vi "启动条件判断.vi"(7 "时间源":T1, 8 "仪器状态":bool, 9 "启动次数":i32, 10 "间隔计时":i32, 11 "周期设置输出":T6={"周期模式"=enum."不启用", "定点周期"={"启动命令"=0, "启动命令 2"=0, "启动命令 3"=0, "启动命令 4"=0, "启动命令 5"=0, "启动命令 6"=0, "启动命令 7"=0, "启动命令 8"=0, "启动命令 9"=0, "启动命令 10"=0, "启动命令 11"=0, "启动命令 12"=0, "启动命令 13"=0, "启动命令 14"=0, "启动命令 15"=0, "启动命令 16"=0, "启动命令 17"=0, "启动命令 18"=0, "启动命令 19"=0, "启动命令 20"=0, "启动命令 21"=0, "启动命令 22"=0, "启动命令 23"=0, "启动命令 24"=0}, "间隔设置"={"启动命令"=0, "启动间隔"=0.0, "启动次数"=0}, "测量参数"={"氨氮"=TRUE, "总磷"=TRUE, "总氮"=TRUE, "CODMn"=TRUE, "CODCr"=TRUE}} {"定点周期"."启动命令 24" items=["", "加标回收（启动采配水）", "加标回收（不启动采配水）", "水样测试（启动采配水）", "水样测试（不启动采配水）"]; "定点周期"."启动命令 23" items=["", "加标回收（启动采配水）", "加标回收（不启动采配水）", "水样测试（启动采配水）", "水样测试（不启动采配水）"]; "定点周期"."启动命令 22" items=["", "加标回收（启动采配水）", "加标回收（不启动采配水）", "水样测试（启动采配水）", "水样测试（不启动采配水）"]; "定点周期"."启动命令 21" items=["", "加标回收（启动采配水）", "加标回收（不启动采配水）", "水样测试（启动采配水）", "水样测试（不启动采配水）"]; "定点周期"."启动命令 20" items=["", "加标回收（启动采配水）", "加标回收（不启动采配水）", "水样测试（启动采配水）", "水样测试（不启动采配水）"]; "定点周期"."启动命令 19" items=["", "加标回收（启动采配水）", "加标回收（不启动采配水）", "水样测试（启动采配水）", "水样测试（不启动采配水）"]; "定点周期"."启动命令 18" items=["", "加标回收（启动采配水）", "加标回收（不启动采配水）", "水样测试（启动采配水）", "水样测试（不启动采配水）"]; "定点周期"."启动命令 17" items=["", "加标回收（启动采配水）", "加标回收（不启动采配水）", "水样测试（启动采配水）", "水样测试（不启动采配水）"]; "定点周期"."启动命令 16" items=["", "加标回收（启动采配水）", "加标回收（不启动采配水）", "水样测试（启动采配水）", "水样测试（不启动采配水）"]; "定点周期"."启动命令 15" items=["", "加标回收（启动采配水）", "加标回收（不启动采配水）", "水样测试（启动采配水）", "水样测试（不启动采配水）"]; "定点周期"."启动命令 14" items=["", "加标回收（启动采配水）", "加标回收（不启动采配水）", "水样测试（启动采配水）", "水样测试（不启动采配水）"]; "定点周期"."启动命令 13" items=["", "加标回收（启动采配水）", "加标回收（不启动采配水）", "水样测试（启动采配水）", "水样测试（不启动采配水）"]; "定点周期"."启动命令 12" items=["", "加标回收（启动采配水）", "加标回收（不启动采配水）", "水样测试（启动采配水）", "水样测试（不启动采配水）"]; "定点周期"."启动命令 11" items=["", "加标回收（启动采配水）", "加标回收（不启动采配水）", "水样测试（启动采配水）", "水样测试（不启动采配水）"]; "定点周期"."启动命令 10" items=["", "加标回收（启动采配水）", "加标回收（不启动采配水）", "水样测试（启动采配水）", "水样测试（不启动采配水）"]; "定点周期"."启动命令 9" items=["", "加标回收（启动采配水）", "加标回收（不启动采配水）", "水样测试（启动采配水）", "水样测试（不启动采配水）"]; "定点周期"."启动命令 8" items=["", "加标回收（启动采配水）", "加标回收（不启动采配水）", "水样测试（启动采配水）", "水样测试（不启动采配水）"]; "定点周期"."启动命令 7" items=["", "加标回收（启动采配水）", "加标回收（不启动采配水）", "水样测试（启动采配水）", "水样测试（不启动采配水）"]; "定点周期"."启动命令 6" items=["", "加标回收（启动采配水）", "加标回收（不启动采配水）", "水样测试（启动采配水）", "水样测试（不启动采配水）"]; "定点周期"."启动命令 5" items=["", "加标回收（启动采配水）", "加标回收（不启动采配水）", "水样测试（启动采配水）", "水样测试（不启动采配水）"]; "定点周期"."启动命令 4" items=["", "加标回收（启动采配水）", "加标回收（不启动采配水）", "水样测试（启动采配水）", "水样测试（不启动采配水）"]; "定点周期"."启动命令 3" items=["", "加标回收（启动采配水）", "加标回收（不启动采配水）", "水样测试（启动采配水）", "水样测试（不启动采配水）"]; "定点周期"."启动命令 2" items=["", "加标回收（启动采配水）", "加标回收（不启动采配水）", "水样测试（启动采配水）", "水样测试（不启动采配水）"]; "定点周期"."启动命令" items=["", "加标回收（启动采配水）", "加标回收（不启动采配水）", "水样测试（启动采配水）", "水样测试（不启动采配水）"]; "间隔设置"."启动命令" items=["", "加标回收（启动采配水）", "加标回收（不启动采配水）", "水样测试（启动采配水）", "水样测试（不启动采配水）"]}) -> (2 "重新配置":bool, 3 "Data":T7={"启动"=FALSE, "控制命令"=enum."加标回收（启动采配水）", "测量参数"={"氨氮"=TRUE, "总磷"=TRUE, "总氮"=TRUE, "CODMn"=TRUE, "CODCr"=TRUE}} caption="数据")   [LabVIEW 2016, in "ZK定时设置.xctl"]
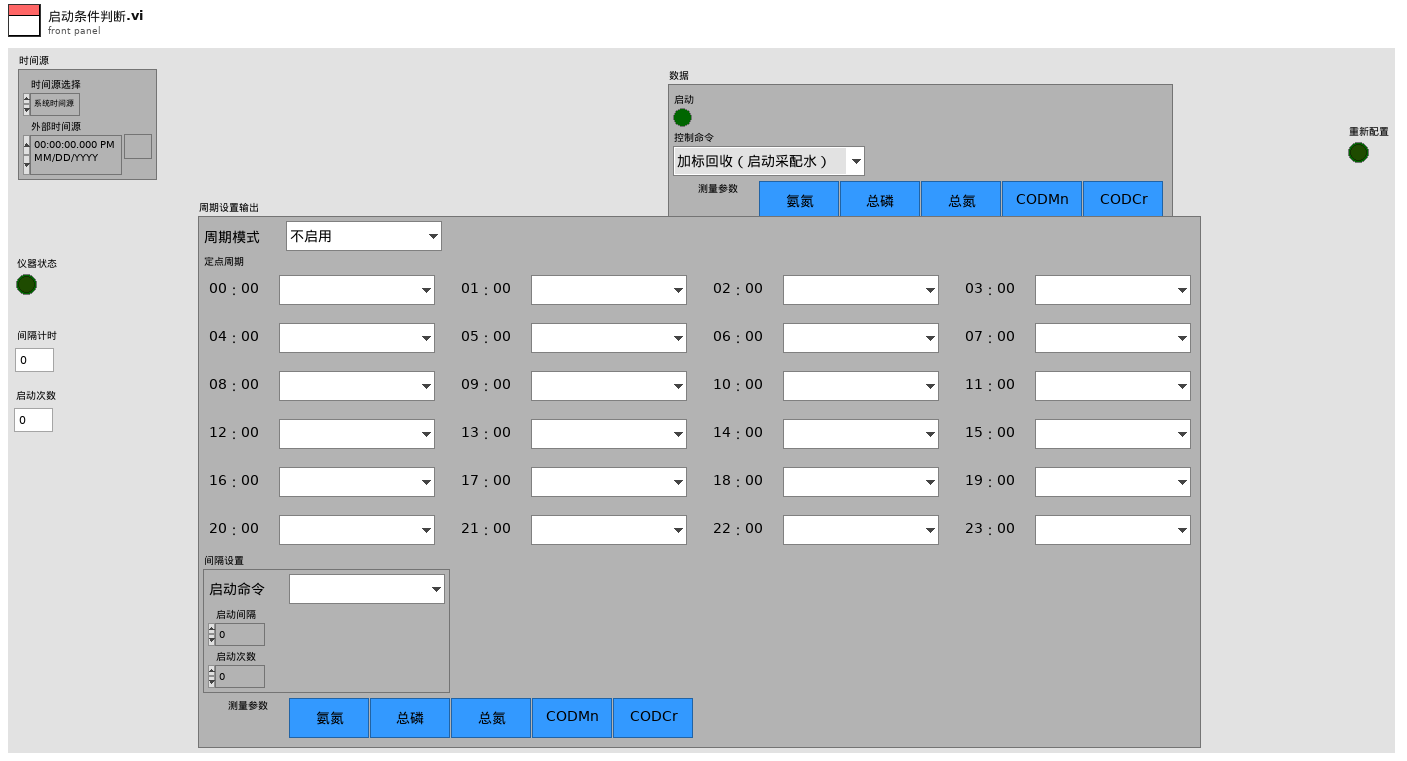
[diagram p1: front panel]
types:
  T1 = cluster{"时间源选择":enum16{"系统时间源", "仪器时间源"}, "外部时间源":timestamp}
  T2 = typedef "ZK定时设置.xctl/周期模式设置.ctl" = enum16{"不启用", "定点模式", "间隔模式"}
  T3 = typedef "ZK定时设置.xctl/定点周期设置.ctl" = cluster{"启动命令":T4, "启动命令 2":T4, "启动命令 3":T4, "启动命令 4":T4, "启动命令 5":T4, "启动命令 6":T4, "启动命令 7":T4, "启动命令 8":T4, "启动命令 9":T4, "启动命令 10":T4, "启动命令 11":T4, "启动命令 12":T4, "启动命令 13":T4, "启动命令 14":T4, "启动命令 15":T4, "启动命令 16":T4, "启动命令 17":T4, "启动命令 18":T4, "启动命令 19":T4, "启动命令 20":T4, "启动命令 21":T4, "启动命令 22":T4, "启动命令 23":T4, "启动命令 24":T4}
  T4 = typedef "ZK定时设置.xctl/启动命令选择.ctl" = u16
  T5 = typedef "ZK定时设置.xctl/测量参数.ctl" = cluster{"氨氮":bool, "总磷":bool, "总氮":bool, "CODMn":bool, "CODCr":bool}
  T6 = cluster{"周期模式":T2, "定点周期":T3, "间隔设置":cluster{"启动命令":T4, "启动间隔":dbl, "启动次数":i32}, "测量参数":T5}
  T7 = typedef "ZK定时设置.xctl/数据.ctl" = cluster{"启动":bool, "控制命令":T8, "测量参数":T5}
  T8 = typedef "ZK定时设置.xctl/国标控制命令.ctl" = enum16{"加标回收（启动采配水）", "加标回收（不启动采配水）", "水样测试（启动采配水）", "水样测试（不启动采配水）"}
  T9 = typedef "LVDateTimeRec.ctl" = cluster{"秒数的小数部分":dbl, "秒":i32, "分":i32, "时":i32, "日":i32, "月":i32, "年":i32, "天数（周）":i32, "天数（年）":i32, "DST":i32}
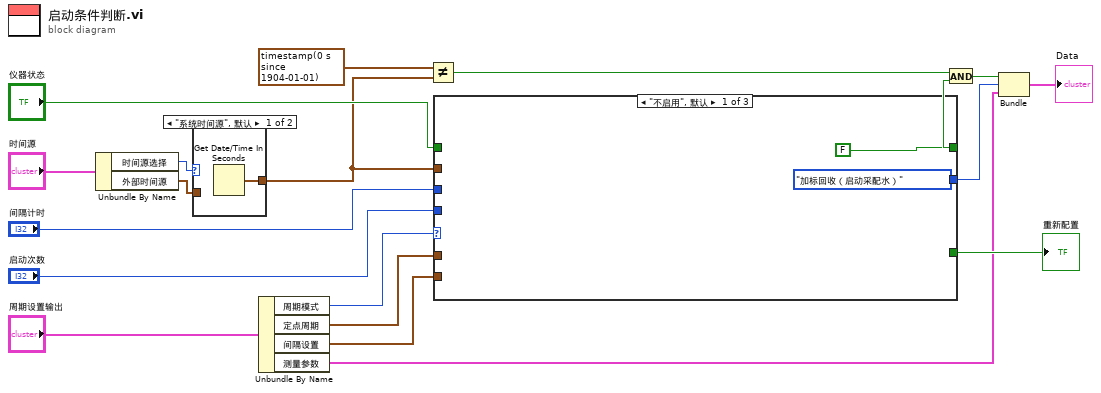
[diagram p0: block diagram]
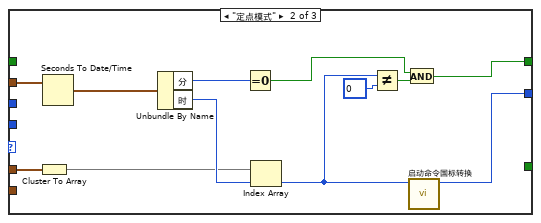
[diagram p3: hidden frame]
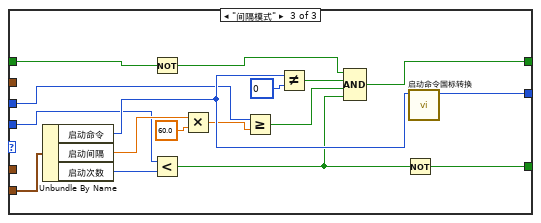
[diagram p4: hidden frame]
diagram:
  n1 = Unbundle By Name("时间源") -> ("时间源选择"=w6:enum16{"系统时间源", "仪器时间源"}, "外部时间源"=w5:timestamp)
  n2 = case shown="\"系统时间源\", 默认" w6 {
    tunnel: [w20 w21] -> w4
    tunnel: w5 -> [_ w21]
    frame "系统时间源", Default {
      n3 = Get Date/Time In Seconds() -> (seconds since 1Jan1904=w20:timestamp)
    }
    frame "仪器时间源" {
    }
  }
  n4 = Unbundle By Name("周期设置输出") -> ("周期模式"=w19:T2, "定点周期"=w18:T3, "间隔设置"=w17:cluster{"启动命令":T4, "启动间隔":dbl, "启动次数":i32}, "测量参数"=w8:T5)
  n5 = Not Equal?(x=timestamp(0 s since 1904-01-01), y=w4) -> (x != y?=w1:bool)
  n6 = case shown="\"不启用\", 默认" w19 {
    tunnel: w18 -> [_ w26 _]
    tunnel: w17 -> [_ _ w52]
    tunnel: [国标控制命令."加标回收（启动采配水）" ("控制命令") w28 w51] -> w15
    tunnel: [FALSE w27 w42] -> w10
    tunnel: "启动次数" -> [_ _ w46]
    tunnel: "间隔计时" -> [_ _ w40]
    tunnel: "仪器状态" -> [_ _ w39]
    tunnel: [_ _ w36] -> w9
    tunnel: w4 -> [_ w24 _]
    frame "不启用", Default {
    }
    frame "定点模式" {
      w33 = T4 0 items=["", "水样测试", "标样核查", "零点核查", "跨度核查", "空白测试", "平行样测试", "加标回收", "空白校准", "标样校准"] ("y")
      n7 = Cluster To Array(cluster=w26) -> (array=w25:T4[])
      n8 = Seconds To Date/Time(time stamp (now)=w24) -> (date time rec=w35:T9)  [unwired: 1 in]
      n9 = Unbundle By Name(w35) -> ("分"=w32:i32, "时"=w34:i32)
      n10 = Equal To 0?(x=w32) -> (x = 0?=w30:bool)
      n11 = Index Array(array=w25, index=w34) -> (element=w29:T4)
      n12 = Not Equal?(x=w29, y=w33) -> (x != y?=w31:bool)
      n13 = And(x=w30, y=w31) -> (x .and. y?=w27:bool)
      n14 = call "启动命令国标转换.vi"("启动命令"=w29) -> ("控制命令"=w28:T8)  [unwired: 10 in]
    }
    frame "间隔模式" {
      w49 = T4 0 items=["", "水样测试", "标样核查", "零点核查", "跨度核查", "空白测试", "平行样测试", "加标回收", "空白校准", "标样校准"] ("y")
      n15 = Unbundle By Name(w52) -> ("启动命令"=w50:T4, "启动间隔"=w48:dbl, "启动次数"=w45:i32)
      n16 = Not(x=w39) -> (.not. x?=w38:bool)
      n17 = Less?(x=w46, y=w45) -> (x < y?=w37:bool)
      n18 = Multiply(x=w48, y=60.0) -> (x*y=w41:dbl)
      n19 = Greater Or Equal?(x=w40, y=w41) -> (x >= y?=w43:bool)
      n20 = Not Equal?(x=w50, y=w49) -> (x != y?=w44:bool)
      n21 = Compound Arithmetic op=AND ("复合运算")(w38, w44, w43, w37) -> (w42:bool)
      n22 = Not(x=w37) -> (.not. x?=w36:bool)
      n23 = call "启动命令国标转换.vi"("启动命令"=w50) -> ("控制命令"=w51:T8)  [unwired: 10 in]
    }
  }
  "重新配置" <- w9
  n24 = And(x=w1, y=w10) -> (x .and. y?=w2:bool)
  n25 = Bundle(w2, "控制命令"=w15, "测量参数"=w8) -> (→"Data":cluster{bool, "控制命令":T8, "测量参数":T5})  [unwired: 1 in]
